vi "CR-纤维毛发检测1处理函数.vi"(8 "error in (no error)":errorcluster caption="错误输入（无错误）", 10 "UI电源线正面漏线参数":T2={"Curve Extraction Settings "={"Extraction Mode"=0, "Edge Threshold"=25, "Edge Filter Size"=1, "Min Length"=19, "Row Search Step Size"=5, "Col Search Step Size"=5, "Max Endpoint Gap"=10, "Closed"=FALSE, "Subpixel"=FALSE}, "Color Mode (Histogram 1)"=0, "Range (Threshold 1)"={"Lower value"=62.0, "Upper value"=255.0}, "Clamp Settings (Max Clamp 1)"={"Angle Range (+/-)"=10.0, "Edge Polarity"={"Start"=0, "End"=0}}, "Settings (Clamp (Rake) 1)"={"Contrast"=6, "Filter width"=5, "Steepness"=2, "Subsampling Ratio"=5, "Show Search Area"=TRUE, "Show Search Lines"=TRUE, "Show Edges Found"=TRUE, "Show Result"=TRUE}, "直径设定"={"Lower value"=62.0, "Upper value"=255.0}} {"Clamp Settings (Max Clamp 1)"."Edge Polarity"."Start" items=["Any", "Rising", "Falling"]; "Clamp Settings (Max Clamp 1)"."Edge Polarity"."End" items=["Any", "Rising", "Falling"]; "Color Mode (Histogram 1)" items=["RGB", "HSL", "HSV", "HSI"]; "Curve Extraction Settings"."Extraction Mode" items=["Normal", "Uniform Regions"]; "Curve Extraction Settings"."Edge Filter Size" items=["Fine", "Normal", "Contour Tracing"]; "Curve Extraction Settings"."Max Endpoint Gap" min=0; "Curve Extraction Settings"."Col Search Step Size" min=1 max=255 step=1; "Curve Extraction Settings"."Row Search Step Size" min=1 max=255 step=1; "Curve Extraction Settings"."Min Length" min=0; "Curve Extraction Settings"."Edge Threshold" min=1 max=350 step=1}, 11 "Image in":T3(plugin-control)) -> (0 "error out":errorcluster caption="错误输出", 1 "纤维毛发":bool, 2 "Distance (Clamp (Rake) 1)":sgl format="%.2f", 3 "Image out":T3(plugin-control), 4 "Edge Coordinates (calibrated) (Clamp (Rake) 1)":cluster{"X":sgl, "Y":sgl}[](array[cluster]) {"Y" format="%.2f"; "X" format="%.2f"})   [LabVIEW 2017]
uses:
  <vilib>/vision/Pattern Matching.llb/IMAQ Curve Parameters.ctl
panel:
  out "x/y":dbl
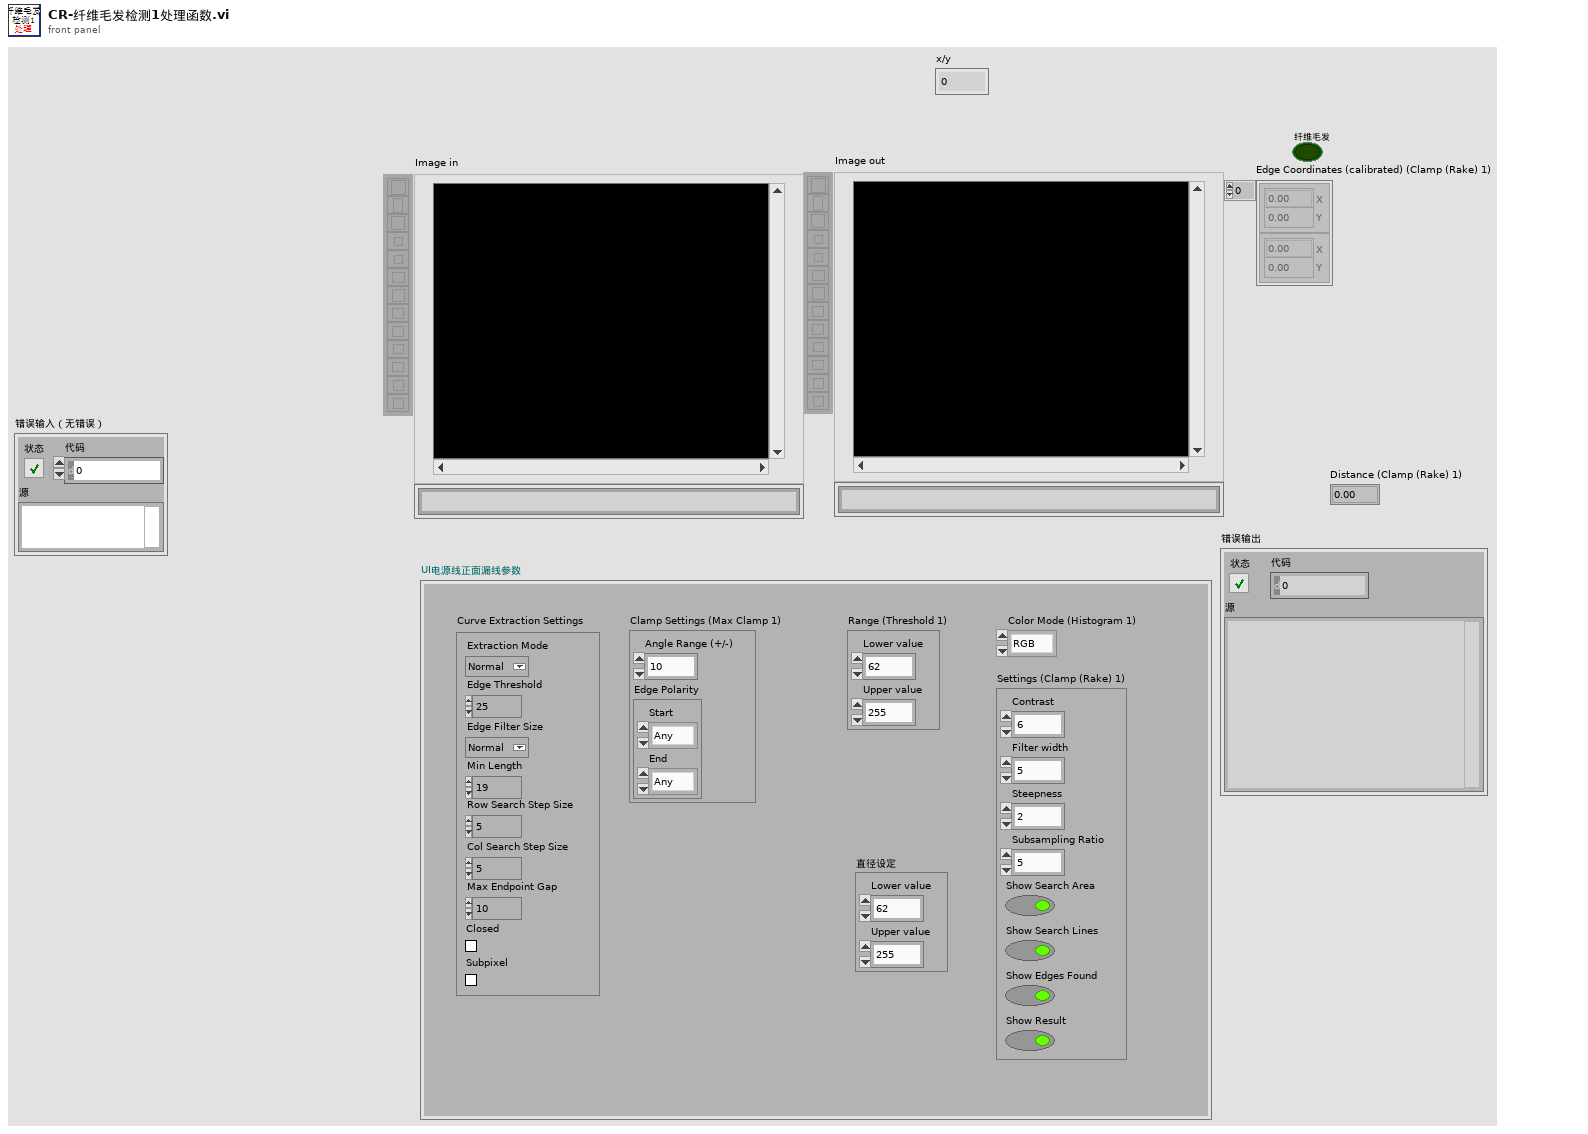
[diagram p1: front panel]
types:
  T1 = typedef "IMAQ Curve Parameters.ctl" = cluster{"Extraction Mode":u32, "Edge Threshold":i32, "Edge Filter Size":u32, "Min Length":i32, "Row Search Step Size":i32, "Col Search Step Size":i32, "Max Endpoint Gap":i32, "Closed":bool, "Subpixel":bool}
  T2 = cluster{"Curve Extraction Settings ":T1, "Color Mode (Histogram 1)":u16, "Range (Threshold 1)":cluster{"Lower value":sgl, "Upper value":sgl}, "Clamp Settings (Max Clamp 1)":cluster{"Angle Range (+/-)":dbl, "Edge Polarity":cluster{"Start":u32, "End":u32}}, "Settings (Clamp (Rake) 1)":cluster{"Contrast":i32, "Filter width":i32, "Steepness":i32, "Subsampling Ratio":u32, "Show Search Area":bool, "Show Search Lines":bool, "Show Edges Found":bool, "Show Result":bool}, "直径设定":cluster{"Lower value":sgl, "Upper value":sgl}}
  T3 = typedef "IMAQ Image.ctl" = refnum<image>
  T4 = cluster{"Contrast":i32, "Filter width":i32, "Steepness":i32, "Subsampling Ratio":u32, "Show Search Area":bool, "Show Search Lines":bool, "Show Edges Found":bool, "Show Result":bool}
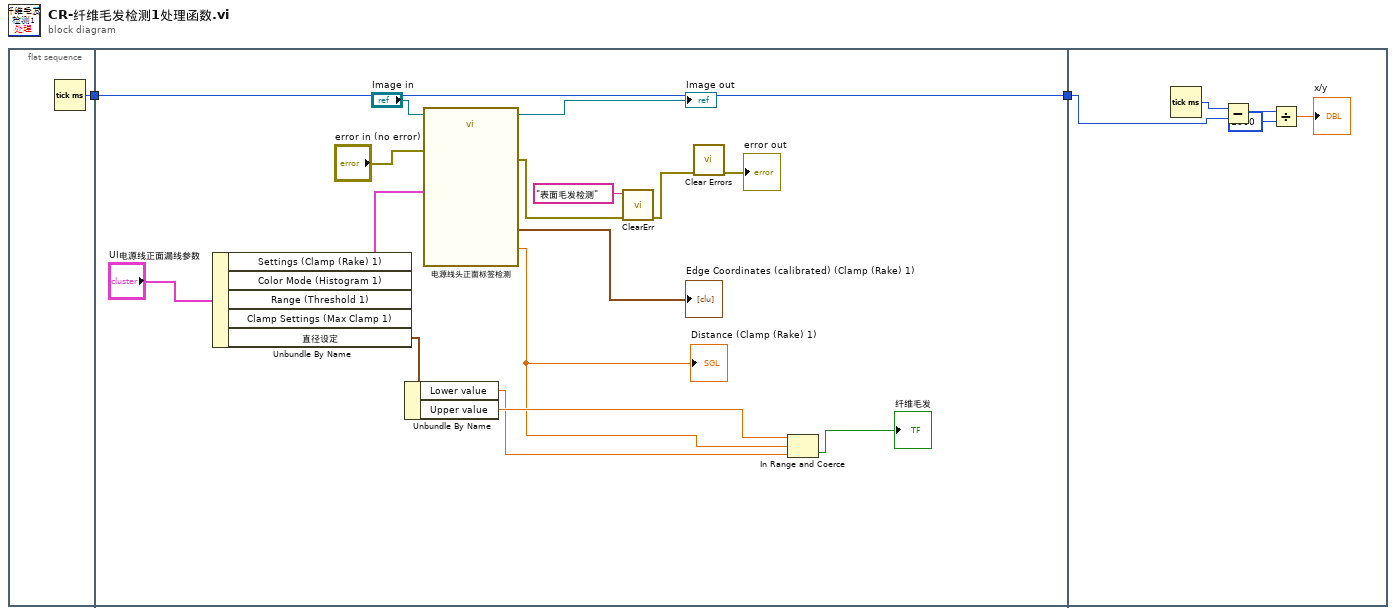
[diagram p0: block diagram]
diagram:
  n1 = flat-sequence {
    tunnel: [w3] -> w1
    tunnel: [w12] -> w2
    tunnel: w1 -> [w12]
    tunnel: w2 -> [w23]
    frame #0 {
      n2 = Tick Count (ms)() -> (millisecond timer value=w3:u32)
    }
    frame #1 {
      n3 = Unbundle By Name("UI电源线正面漏线参数") -> ("Settings (Clamp (Rake) 1)"=w16:T4, "直径设定"=w7:cluster{"Lower value":sgl, "Upper value":sgl})  [unwired: 3 out]
      n4 = Unbundle By Name(w7) -> ("Lower value"=w5:sgl, "Upper value"=w6:sgl)
      n5 = call "电源线头正面标签检测"("Image In"="Image in", "Settings (Clamp (Rake) 1)"=w16, "error in"="error in (no error)") -> ("Image Out"=→"Image out":T3, "Distance (Clamp (Rake) 1)"=w4:sgl, "Edge Coordinates (calibrated) (Clamp (Rake) 1)"=→"Edge Coordinates (calibrated) (Clamp (Rake) 1)":cluster{"X":sgl, "Y":sgl}[], "error out"=w10:errorcluster)  [unwired: 21 in]
      "Distance (Clamp (Rake) 1)" <- w4
      n6 = call "ClearErr.vi"("error in (no error)"=w10, "运行位置"="表面毛发检测") -> ("error out"=w9:errorcluster)  [unwired: 9 in]
      n7 = call <vilib>:"Clear Errors.vi"("error in (no error)"=w9) -> ("error out"=→"error out":errorcluster)  [unwired: 5 in, 1 out]
      n8 = In Range and Coerce(upper limit=w6, x=w4, lower limit=w5) -> (In Range?=→"纤维毛发":bool)  [unwired: 1 out]
    }
    frame #2 {
      n9 = Tick Count (ms)() -> (millisecond timer value=w24:u32)
      n10 = Subtract(x=w24, y=w23) -> (x-y=w22:u32)
      n11 = Divide(x=w22, y=u32 1000) -> (x/y=→"x/y":dbl)
    }
  }
